vi "Is bank data ready.vi"(8 "error IO":errorcluster, 11 "OPC connections":T1) -> (0 "error out":errorcluster, 3 "OPC connections out":T1, 4 "Data ready":bool)   [LabVIEW 2015]
uses:
  OPC connections.ctl
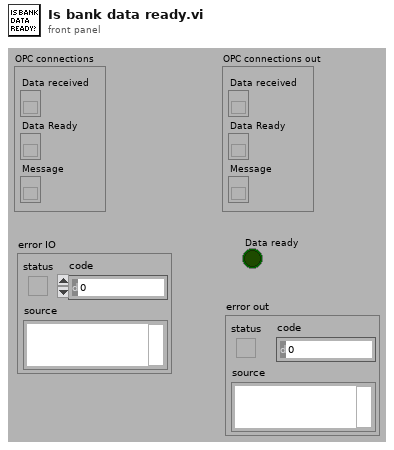
[diagram p1: front panel]
types:
  T1 = typedef "OPC connections.ctl" = cluster{"Data received":refnum<k13>, "Data Ready":refnum<k13>, "Message":refnum<k13>}
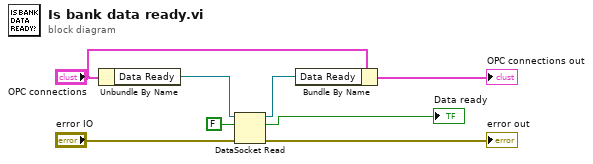
[diagram p0: block diagram]
diagram:
  n1 = Unbundle By Name("OPC connections") -> ("Data Ready"=w5:refnum<k13>)
  n2 = DataSocket Read(8:"error IO", 10:FALSE, 11:w5) -> (0:→"error out":errorcluster, 2:→"Data ready":bool, 3:w7:refnum<k13>)  [unwired: 2 in, 4 out]
  n3 = Bundle By Name(cluster="OPC connections", "Data Ready"=w7) -> (→"OPC connections out":T1)
